vi "PUT-POST Request.vi"(7 "Request":T1=enum."PUT", 8 "error in (no error)":errorcluster, 9 "Request Payload":string, 10 "Path (after URL)":string, 11 "EnVision REST in":refnum<class "EnVision REST.lvclass">) -> (0 "error out":errorcluster, 1 "Status Code":u16, 2 "Response":string, 3 "EnVision REST out":refnum<class "EnVision REST.lvclass">)   [LabVIEW 2018, in "EnVision REST.lvlib" / "EnVision REST.lvclass"]
uses:
  EnVision REST.lvclass
  PPLs/REST Interface/Parent/REST Interface.lvlibp/Custom Controls/Request.ctl
  EnVision REST.lvclass/EnVision REST.ctl
  <vilib>/addons/_JKI.lib/REST Client/classes/REST Client/REST Client.lvclass
  PPLs/REST Interface/Parent/REST Interface.lvlibp/REST Interface.lvclass
  C:/Projects/LabVIEW/PPLs/REST Interface/Parent/REST Interface.lvlibp/REST Interface.lvclass
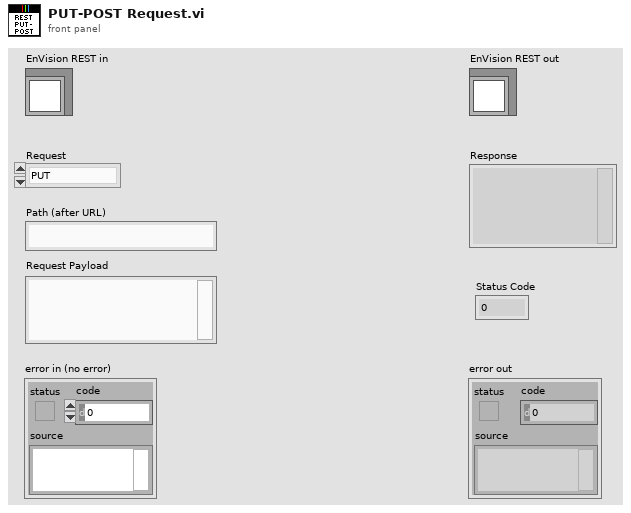
[diagram p1: front panel]
types:
  T1 = typedef "REST Interface.lvlibp/REST Interface.lvclass/Request.ctl" = enum16{"HEAD", "PUT", "GET", "POST", "DELETE"}
  T2 = typedef "REST Interface.lvlibp/REST Client.lvlib/REST Client.lvclass/HTTP Header.ctl" = cluster{"header":string, "value":string}
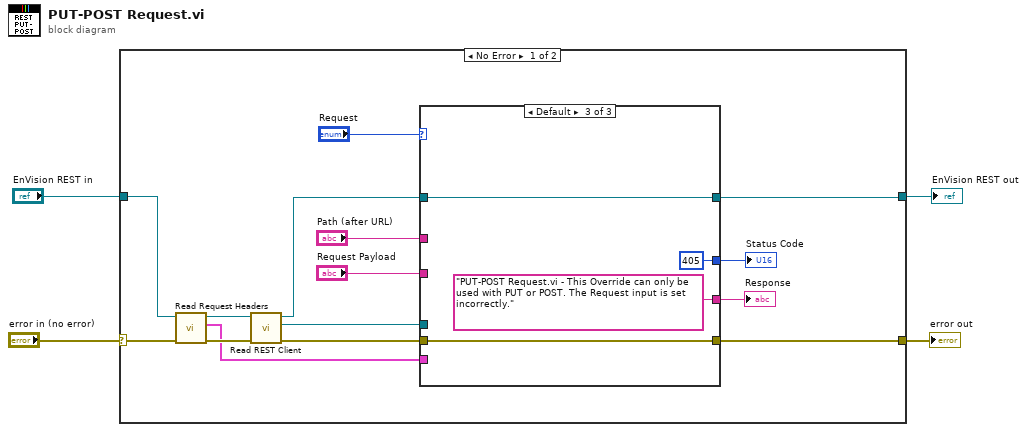
[diagram p0: block diagram]
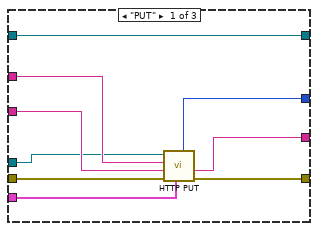
[diagram p2: hidden frame]
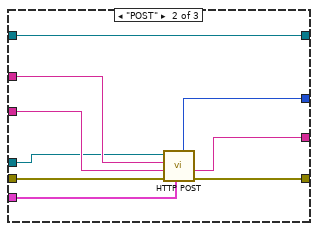
[diagram p3: hidden frame]
diagram:
  n1 = case shown="No Error" "error in (no error)" {
    selector: "error in (no error)" -> [w7 w43]
    tunnel: [w14 w43] -> w3
    tunnel: [w17 w42] -> w2
    tunnel: "EnVision REST in" -> [w9 w42]
    frame No Error {
      n2 = call "Read Request Headers.vi"("error in (no error)"=w7, "REST Interface in"=w9) -> ("error out"=w6:errorcluster, "Request Headers"=w5:T2[], "REST Interface out"=w8:refnum<class "EnVision REST.lvclass">)  [unwired: 7 in]
      n3 = call "Read REST Client.vi"("error in (no error)"=w6, "EnVision REST in"=w8) -> ("error out"=w15:errorcluster, "REST Client.lvlib:REST Client.lvclass"=w16:refnum<class "REST Client.lvclass">, "EnVision REST out"=w18:refnum<class "EnVision REST.lvclass">)  [unwired: 7 in]
      n4 = case shown="Default" "Request" {
        tunnel: w18 -> [w28 w37 w41]
        tunnel: [w28 w37 w41] -> w17
        tunnel: w16 -> [w21 w30 _]
        tunnel: w15 -> [w27 w36 w38]
        tunnel: [w26 w35 w38] -> w14
        tunnel: [w25 w34 u16 405 ("Status Code")] -> w13
        tunnel: [w24 w33 "PUT-POST Request.vi - This Override can only be used with PUT or POST. The Request input is set incorrectly." ("Response body")] -> w12
        tunnel: "Path (after URL)" -> [w23 w32 _]
        tunnel: "Request Payload" -> [w22 w31 _]
        tunnel: w5 -> [w20 w29 _]
        frame "PUT" {
          n5 = call-dynamic "HTTP PUT.vi"("request specific headers"=w20, "error in (no error)"=w27, "Request body"=w22, "Path"=w23, "REST Client in"=w21) -> ("error out"=w26:errorcluster, "Response body"=w24:string, "Status Code"=w25:u16)  [unwired: 1 in, 3 out]
        }
        frame "POST" {
          n6 = call-dynamic "HTTP POST.vi"("request specific headers"=w29, "error in (no error)"=w36, "Request body"=w31, "Path"=w32, "REST Client in"=w30) -> ("error out"=w35:errorcluster, "Response body"=w33:string, "Status Code"=w34:u16)  [unwired: 1 in, 3 out]
        }
        frame Default {
        }
      }
      "Status Code" <- w13
      "Response" <- w12
    }
    frame Error {
    }
  }
  "error out" <- w3
  "EnVision REST out" <- w2
